vi "ProjetAsserv.vi"() -> ()   [LabVIEW 2021]
uses:
  <vilib>/MakerHub/LINX/Public/Peripherals/Analog/Analog Read 1 Chan.vi
  <vilib>/MakerHub/LINX/Public/Peripherals/PWM/PWM Set Duty Cycle 1 Chan.vi
  <vilib>/MakerHub/LINX/Public/Peripherals/Analog/Analog Read N Chans.vi
  <vilib>/MakerHub/LINX/Private/Local IO/LinxAnalogRead.vi
  <vilib>/MakerHub/LINX/Public/Utilities/Check Channel.vi
  <vilib>/MakerHub/LINX/Public/Utilities/Open Serial.vi
  <vilib>/MakerHub/LINX/Private/Utilties/Generate Error.vi
  <vilib>/MakerHub/LINX/Public/Peripherals/PWM/PWM Set Duty Cycle N Chans.vi
  <vilib>/MakerHub/LINX/LMH-LINX.lvlib
panel:
  in  "Stop Button":bool
  out "V/3.3":dbl
  out "Voltage":dbl
  in  "Analog Pin":u8=3
  in  "Serial Port 3":refnum<visa-resource-name>
  in  "PWM Pin":u8=3
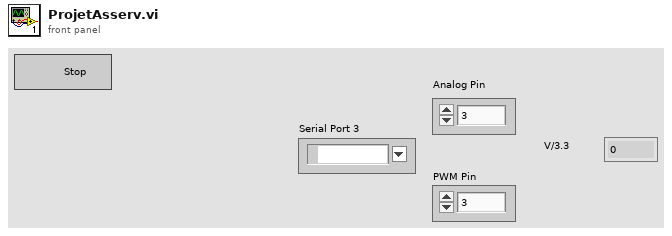
[diagram p1: front panel]
types:
  T1 = typedef "LMH-LINX.lvlib/LINX Ref.ctl" = cluster{"IO":T2, "Interface":T3, "LINX Device Config":T4}
  T2 = typedef "LMH-LINX.lvlib/Platform.ctl" = enum16{"Remote", "Local"}
  T3 = typedef "LMH-LINX.lvlib/Interface.ctl" = enum16{"Serial", "TCP"}
  T4 = typedef "LMH-LINX.lvlib/Device.lvlib/LINX Device Config.ctl" = cluster{"Interface":T3, "COM Port":refnum<visa-resource-name>, "TCP Configuration":T5, "Device Family":u8, "Device ID":u8, "Device Name":string, "TCP Ref":refnum<k5>, "Channels":T6}
  T5 = typedef "LMH-LINX.lvlib/Device.lvlib/TCP Config.ctl" = cluster{"IP Address":string, "Port":u16}
  T6 = typedef "LMH-LINX.lvlib/Channels.ctl" = cluster{"DI":u8[], "DO":u8[], "AI":u8[], "AO":u8[], "PWM":u8[], "QE":u8[], "UART":u8[], "I2C 2":u8[], "SPI":u8[], "CAN":u8[], "Servo":u8[], "AI Ref (V)":dbl, "AI Resolution (Bits)":u8, "AO Ref (V)":dbl, "AO Resolution (Bits)":u8}
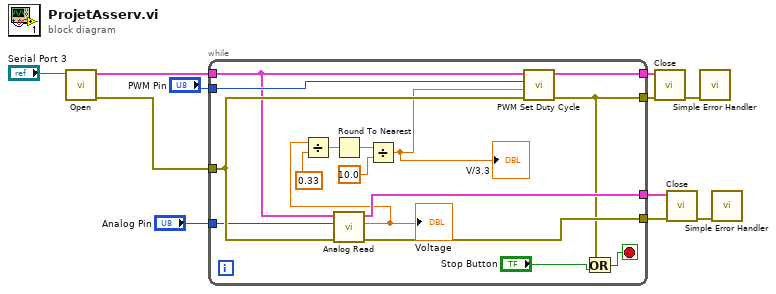
[diagram p0: block diagram]
diagram:
  n1 = call-poly <vilib>:"Open.vi"("Serial Port"="Serial Port 3") -> ("Error Out"=w9:errorcluster, "LINX Resource"=w5:T1)  [unwired: 8 in, 1 out]
  n2 = while {
    tunnel: "PWM Pin" -> [w26]
    tunnel: w9 -> [w25]
    tunnel: [w14] -> w7
    tunnel: [w27] -> w6
    tunnel: w5 -> [w23]
    tunnel: "Analog Pin" -> [w24]
    tunnel: [w22] -> w2
    tunnel: [w21] -> w1
    stop <- w12 stop-if-true
    n3 = call-poly <vilib>:"Analog Read.vi"("Error In"=w25, "Analog Channel"=w24, "LINX Resource"=w23) -> ("Error Out"=w21:errorcluster, "Voltage"=w20:dbl, "LINX Resource"=w22:T1)  [unwired: 5 in, 1 out]
    "Voltage" <- w20
    n4 = Divide(x=w20, y=0.33) -> (x/y=w18:dbl)
    n5 = Round To Nearest(number=w18) -> (nearest integer value=w17:dbl)
    n6 = Divide(x=w17, y=10.0) -> (x/y=w15:dbl)
    "V/3.3" <- w15
    n7 = call-poly <vilib>:"PWM Set Duty Cycle.vi"("Error In"=w25, "Duty Cycle (0-1)"=w15, "PWM Channel"=w26, "LINX Resource"=w23) -> ("Error Out"=w14:errorcluster, "LINX Resource"=w27:T1)  [unwired: 6 in]
    n8 = Or(x=w14, y="Stop Button") -> (x .or. y?=w12:bool)
  }
  n9 = call <vilib>:"Close.vi"("Error In"=w7, "LINX Resource"=w6) -> ("Error Out"=w8:errorcluster)  [unwired: 9 in]
  n10 = call <vilib>:"Close.vi"("Error In"=w1, "LINX Resource"=w2) -> ("Error Out"=w3:errorcluster)  [unwired: 9 in]
  n11 = call <vilib>:"Simple Error Handler.vi"("error in (no error)"=w8) -> ()  [unwired: 4 in, 5 out]
  n12 = call <vilib>:"Simple Error Handler.vi"("error in (no error)"=w3) -> ()  [unwired: 4 in, 5 out]
